vi "Parse KLS_Query type answer by type.vi"(0 "KLS? response":string, 1 "Type":string, 5 "error in (no error)":errorcluster) -> (14 "Names":string[](array[string]), 19 "error out":errorcluster)   [LabVIEW 2020]
doc: "Filters the response of KLS? type answers by the selected type and returns all names related to that type."
uses:
  Match Regular Expression.xnode
panel:
  # "Filters the response of KLS? type answers by the selected type\nand returns all names related to that type."
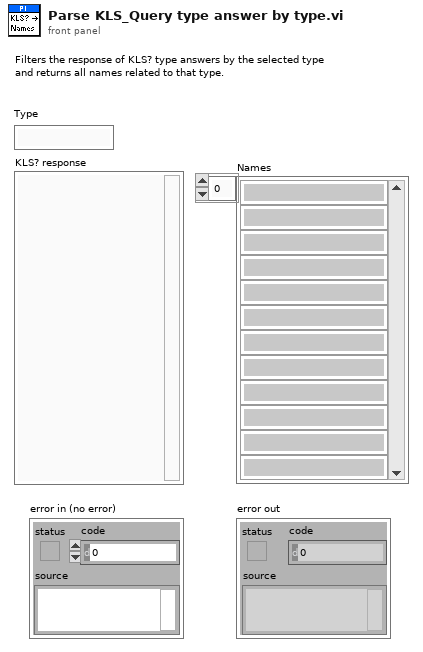
[diagram p1: front panel]
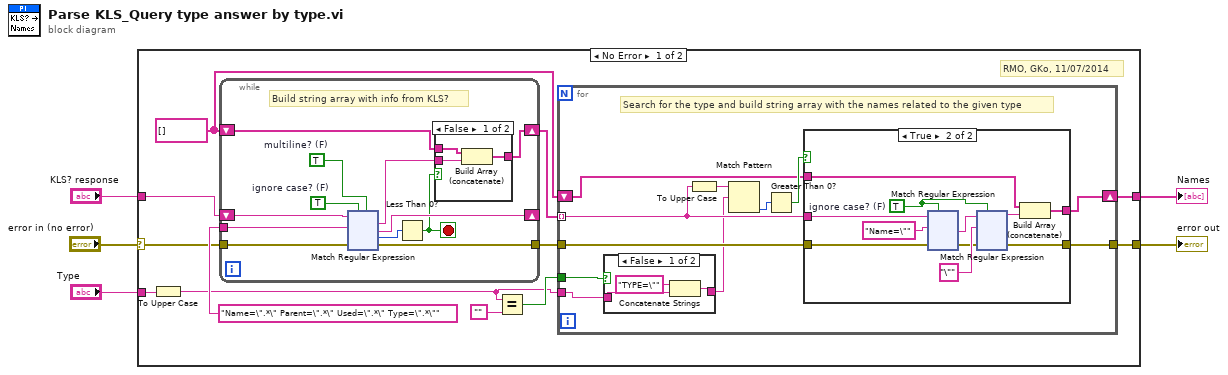
[diagram p0: block diagram]
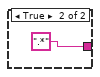
[diagram p2: hidden frame]
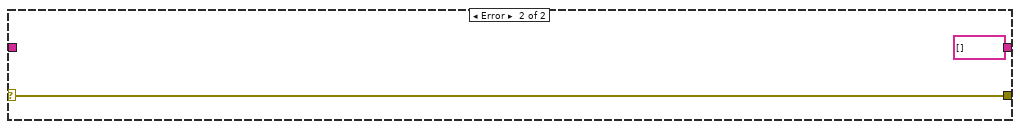
[diagram p5: hidden frame]
diagram:
  n1 = case shown="No Error" "error in (no error)" {
    selector: "error in (no error)" -> [w12 w405]
    tunnel: [w15 string[] []] -> w5
    tunnel: "KLS? response" -> [w13 _]
    tunnel: [w10 w405] -> w3
    tunnel: "Type" -> [w7 _]
    frame No Error {
      w14 = string[] []
      # "RMO, GKo, 11/07/2014"
      n2 = To Upper Case(1:w7) -> (0:w6:string)
      n3 = while {
        shift-right: [w280] -> _
        shift-left: w13 -> [w283]
        tunnel: "Name=\".*\" Parent=\".*\" Used=\".*\" Type=\".*\"" -> [w277]
        shift-right: [w279] -> w16
        shift-left: w14 -> [w282]
        tunnel: w12 -> [w275]
        tunnel: [w274] -> w11
        stop <- w276 stop-if-true
        w285 = TRUE  # ignore case? (F)
        w284 = TRUE  # multiline? (F)
        # "Build string array with info from KLS?"
        n4 = xnode "Match Regular Expression"("input string"=w283, "regular expression"=w277, "error in"=w275, "ignore case? (F)"=w285, "multiline? (F)"=w284) -> ("whole match"=w281:string, "after match"=w280:string, "offset past match"=w278:i32, "error out"=w274:errorcluster)  [unwired: 1 in, 1 out]
        n5 = Less Than 0?(x=w278) -> (x < 0?=w276:bool)
        n6 = case shown="False" w276 {
          tunnel: w282 -> [w288 w289]
          tunnel: w281 -> [w287 _]
          tunnel: [w286 w289] -> w279
          frame False {
            n7 = Build Array (concatenate)(w288, w287) -> (w286:string[])
          }
          frame True {
          }
        }
      }
      n8 = Equal?(x=w6, y="") -> (x = y?=w9:bool)
      n9 = for {
        tunnel: w16 -> [w22] mode=indexing
        shift-right: [w25] -> w15
        shift-left: w14 -> [w26]
        tunnel: w11 -> [w24]
        tunnel: [w23] -> w10
        tunnel: w9 -> [w19]
        tunnel: w6 -> [w18]
        # "Search for the type and build string array with the names related to the given type"
        n10 = case shown="False" w19 {
          tunnel: [w29 ".*"] -> w20
          tunnel: w18 -> [w30 _]
          frame False {
            n11 = Concatenate Strings("TYPE=\"", w30) -> (w29:string)
          }
          frame True {
          }
        }
        n12 = To Upper Case(1:w22) -> (0:w21:string)
        n13 = Match Pattern(string=w21, regular expression=w20) -> (offset past match=w28:i32)  [unwired: 4 out]
        n14 = Greater Than 0?(x=w28) -> (x > 0?=w27:bool)
        n15 = case shown="True" w27 {
          tunnel: w22 -> [_ w41]
          tunnel: w26 -> [w34 w40]
          tunnel: [w34 w38] -> w25
          tunnel: w24 -> [w33 w37]
          tunnel: [w33 w35] -> w23
          frame False {
          }
          frame True {
            w44 = TRUE  # ignore case? (F)
            n16 = xnode "Match Regular Expression"("input string"=w41, "regular expression"="Name=\"", "error in"=w37, "ignore case? (F)"=w44) -> ("after match"=w42:string, "error out"=w36:errorcluster)  [unwired: 1 in, 4 out]
            n17 = xnode "Match Regular Expression"("input string"=w42, "regular expression"="\"", "error in"=w36, "ignore case? (F)"=w44) -> ("before match"=w39:string, "error out"=w35:errorcluster)  [unwired: 1 in, 4 out]
            n18 = Build Array (concatenate)(w40, w39) -> (w38:string[])
          }
        }
      }
    }
    frame Error {
    }
  }
  "Names" <- w5
  "error out" <- w3
